vi "Log Final Process Error.vi"(8 "error in (no error)":errorcluster, 10 "Trace":refnum<class "RequestTraceLog.lvclass">, 11 "Server in":refnum<class "Server.lvclass">) -> (0 "error out":errorcluster, 3 "Server out":refnum<class "Server.lvclass">)   [LabVIEW 2020, in "HTTP Server.lvlib" / "Server.lvclass"]
uses:
  Server.lvclass
  Server.lvclass/Server.ctl
  RequestTraceLog/RequestTraceLog.lvclass
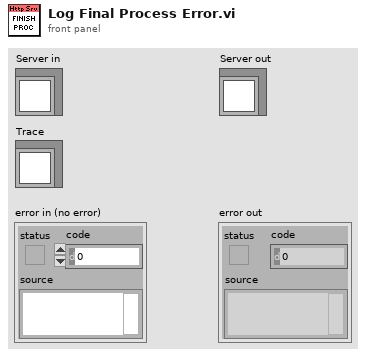
[diagram p1: front panel]
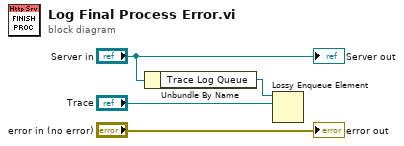
[diagram p0: block diagram]
diagram:
  n1 = Unbundle By Name("Server in") -> ("Trace Log Queue"=w2:refnum<queue>)
  n2 = Lossy Enqueue Element(queue=w2, element="Trace") -> ()  [unwired: 1 in, 4 out]
  "error out" <- "error in (no error)"
  "Server out" <- "Server in"
